vi "Rohde & Schwarz VNA Set Stimulus.vi"(7 "Rohde & Schwarz VNA":T4={"Model"="8753C", "Serial"="", "Firmware"="", "Setup File"=""}, 8 "error in (no error)":errorcluster, 9 "Channel":i8=1 min=1 max=99 step=1, 10 "Stimulus":T1={"Use Instrument Settings"=FALSE, "Blank Frequencies"=FALSE, "Sweep Type"=enum."Linear", "Sweep"={"Fstart"=500.0, "Fstop"=1500.0, "Units"=enum."MHz", "Points"=201}, "Power (dBm)"=999.0, "IFBW (Hz)"=-1.0, "Sweep Time (s)"=-1.0, "Calibration"={"State"=FALSE, "String"=""}} {"Sweep Time (s)" format="%.3g"}, 11 "VISA Resource Name":refnum<visa-resource-name>) -> (0 "error out":errorcluster {"code" format="%.0x"}, 3 "dup VISA Resource Name":refnum<visa-resource-name>)   [LabVIEW 2011]
uses:
  TypeDefs/Rohde & Schwarz VNA Instrument Info.ctl
  tests/S Parameter/TypeDefs/SP Stimulus Parameters.ctl
  tests/S Parameter/TypeDefs/SP Frequency Units.ctl
  tests/S Parameter/TypeDefs/SP Calibration State.ctl
  TypeDefs/Rohde & Schwarz VNA Sweep Type.ctl
  TypeDefs/Rohde & Schwarz VNA Trigger Mode.ctl
panel:
  in  "Case Constant\n(See Context Help)":bool
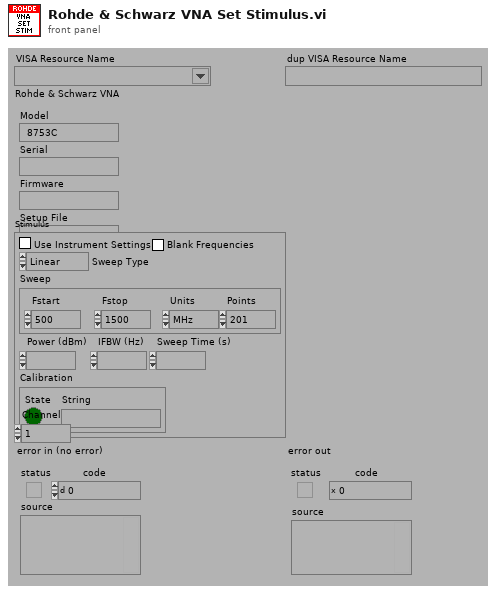
[diagram p1: front panel]
types:
  T1 = typedef "SP Stimulus Parameters.ctl" = cluster{"Use Instrument Settings":bool, "Blank Frequencies":bool, "Sweep Type":enum32{"Linear", "Logarithmic", "List", "Power", "CW"}, "Sweep":cluster{"Fstart":dbl, "Fstop":dbl, "Units":T2, "Points":i32}, "Power (dBm)":dbl, "IFBW (Hz)":dbl, "Sweep Time (s)":dbl, "Calibration":T3}
  T2 = typedef "SP Frequency Units.ctl" = enum16{"Hz", "kHz", "MHz", "GHz", "Points"}
  T3 = typedef "SP Calibration State.ctl" = cluster{"State":bool, "String":string}
  T4 = typedef "Rohde & Schwarz VNA Instrument Info.ctl" = cluster{"Model":string, "Serial":string, "Firmware":string, "Setup File":string}
  T5 = typedef "Rohde & Schwarz VNA Sweep Type.ctl" = enum32{"Linear", "Logarithmic", "Segmented", "Power", "Time", "CW"}
  T6 = typedef "Rohde & Schwarz VNA Trigger Mode.ctl" = enum16{"Continuous", "Hold", "Single"}
  T7 = enum32{"Linear", "Logarithmic", "List", "Power", "CW"}
  T8 = cluster{"Converted Frequency":dbl, "Converted Frequency":dbl}
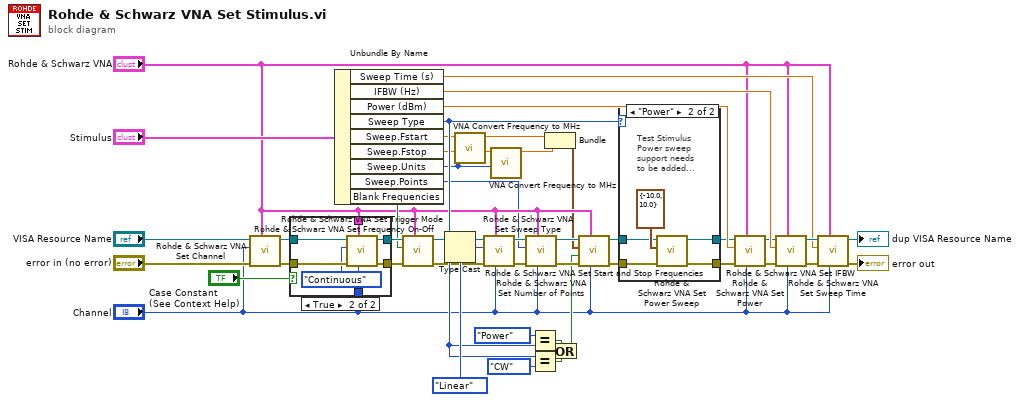
[diagram p0: block diagram]
diagram:
  n1 = call "Rohde & Schwarz VNA Set Channel.vi"("Rohde & Schwarz VNA"="Rohde & Schwarz VNA", "error in (no error)"="error in (no error)", "Channel"="Channel", "VISA Resource Name"="VISA Resource Name") -> ("error out"=w35:errorcluster, "dup VISA Resource Name"=w34:refnum<visa-resource-name>)  [unwired: 6 out]
  n2 = case shown="True" "Case Constant\n(See Context Help)" {
    tunnel: [w47 w51] -> w16
    tunnel: [w46 w52] -> w15
    tunnel: w35 -> [w47 w54]
    tunnel: w34 -> [w46 w53]
    tunnel: "Rohde & Schwarz VNA" -> [_ w49]
    tunnel: "Channel" -> [_ w48]
    frame False {
    }
    frame True {
      n3 = call "Rohde & Schwarz VNA Set Trigger Mode.vi"("Channel"=w48, "Rohde & Schwarz VNA"=w49, "error in (no error)"=w54, "Trigger Mode"=Rohde_&_Schwarz_VNA_Trigger_Mode."Continuous", "VISA Resource Name"=w53) -> ("error out"=w51:errorcluster, "dup VISA Resource Name"=w52:refnum<visa-resource-name>)  [unwired: 5 out]
    }
  }
  n4 = Unbundle By Name("Stimulus") -> ("Sweep Time (s)"=w38:dbl, "IFBW (Hz)"=w43:dbl, "Power (dBm)"=w44:dbl, "Sweep Type"=w19:T7, "Sweep.Fstart"=w6:dbl, "Sweep.Fstop"=w5:dbl, "Sweep.Units"=w4:T2, "Sweep.Points"=w7:i32, "Blank Frequencies"=w12:bool)
  n5 = call "Rohde & Schwarz VNA Set Frequency On-Off.vi"("Rohde & Schwarz VNA"="Rohde & Schwarz VNA", "error in (no error)"=w16, "Blank Frequencies (F)"=w12, "VISA Resource Name"=w15) -> ("error out"=w13:errorcluster, "dup VISA Resource Name"=w14:refnum<visa-resource-name>)  [unwired: 6 out]
  n6 = Type Cast(type=Rohde_&_Schwarz_VNA_Sweep_Type."Linear" ("Sweep Type"), x=w19) -> (*(type *) &x=w30:T5)
  n7 = call "VNA Convert Frequency to MHz.vi"("Units"=w4, "Frequency"=w6) -> ("Converted Frequency"=w2:dbl)  [unwired: 9 out]
  n8 = call "Rohde & Schwarz VNA Set Sweep Type.vi"("Channel"="Channel", "Rohde & Schwarz VNA"="Rohde & Schwarz VNA", "error in (no error)"=w13, "Sweep Type"=w30, "VISA Resource Name"=w14) -> ("error out"=w26:errorcluster, "dup VISA Resource Name"=w27:refnum<visa-resource-name>)  [unwired: 5 out]
  n9 = call "VNA Convert Frequency to MHz.vi"("Units"=w4, "Frequency"=w5) -> ("Converted Frequency"=w1:dbl)  [unwired: 9 out]
  n10 = call "Rohde & Schwarz VNA Set Number of Points.vi"("Channel"="Channel", "Rohde & Schwarz VNA"="Rohde & Schwarz VNA", "error in (no error)"=w26, "Number Points"=w7, "VISA Resource Name"=w27) -> ("error out"=w28:errorcluster, "dup VISA Resource Name"=w29:refnum<visa-resource-name>)  [unwired: 5 out]
  n11 = Equal?(x=enum32{"Linear", "Log", "List", "Power", "CW"}."Power" ("Sweep Type"), y=w19) -> (x = y?=w23:bool)
  n12 = Equal?(x=w19, y=enum32{"Linear", "Log", "List", "Power", "CW"}."CW" ("Sweep Type")) -> (x = y?=w22:bool)
  n13 = Bundle("Converted Frequency"=w2, "Converted Frequency"=w1) -> (w3:T8)  [unwired: 1 out]
  n14 = Or(x=w23, y=w22) -> (x .or. y?=w18:bool)
  n15 = call "Rohde & Schwarz VNA Set Start and Stop Frequencies.vi"("Channel"="Channel", "Rohde & Schwarz VNA"="Rohde & Schwarz VNA", "error in (no error)"=w28, "CW? (f)"=w18, "Start/Stop Freqs, MHz"=w3, "VISA Resource Name"=w29) -> ("error out"=w25:errorcluster, "dup VISA Resource Name"=w24:refnum<visa-resource-name>)  [unwired: 4 out]
  n16 = case shown="\"Power\"" w19 {
    tunnel: w25 -> [w56 w58]
    tunnel: w24 -> [w55 w57]
    tunnel: [w55 w60] -> w42
    tunnel: [w56 w59] -> w41
    frame "Linear", "Logarithmic", "CW", Default {
    }
    frame "Power" {
      # "Test Stimulus\nPower sweep\nsupport needs\nto be added..."
      n17 = call "Rohde & Schwarz VNA Set Power Sweep.vi"("error in (no error)"=w58, "Start/Stop Power, dBm"=cluster{"Pstart":dbl, "Pstop":dbl} {"Pstart"=-10.0, "Pstop"=10.0}, "VISA Resource Name"=w57) -> ("error out"=w59:errorcluster, "dup VISA Resource Name"=w60:refnum<visa-resource-name>)  [unwired: 7 out]
    }
  }
  n18 = call "Rohde & Schwarz VNA Set Power.vi"("Channel"="Channel", "Rohde & Schwarz VNA"="Rohde & Schwarz VNA", "error in (no error)"=w41, "Source Power, dBm (0.0)"=w44, "VISA Resource Name"=w42) -> ("error out"=w37:errorcluster, "dup VISA Resource Name"=w36:refnum<visa-resource-name>)  [unwired: 5 out]
  n19 = call "Rohde & Schwarz VNA Set IFBW.vi"("Channel"="Channel", "Rohde & Schwarz VNA"="Rohde & Schwarz VNA", "error in (no error)"=w37, "IFBW, Hz (3000)"=w43, "VISA Resource Name"=w36) -> ("error out"=w40:errorcluster, "dup VISA Resource Name"=w39:refnum<visa-resource-name>)  [unwired: 5 out]
  n20 = call "Rohde & Schwarz VNA Set Sweep Time.vi"("Channel"="Channel", "Rohde & Schwarz VNA"="Rohde & Schwarz VNA", "error in (no error)"=w40, "Sweep Time, s (-1: Auto)"=w38, "VISA Resource Name"=w39) -> ("error out"=→"error out":errorcluster, "dup VISA Resource Name"=→"dup VISA Resource Name":refnum<visa-resource-name>)  [unwired: 5 out]
